vi "PopulateClearCycles.vi"(10 "ClearCycles":refnum<k24>, 11 "Digital in":refnum<vi>) -> ()   [LabVIEW 2019]
uses:
  Dependencies/PVCamNET.dll
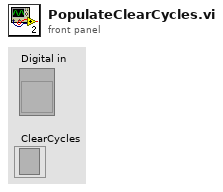
[diagram p1: front panel]
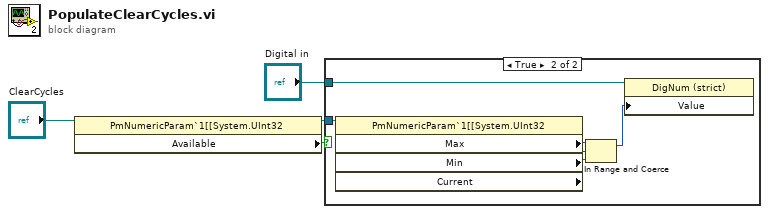
[diagram p0: block diagram]
diagram:
  n1 = property class="PmNumericParam`1[[System.UInt32"(reference="ClearCycles") -> (reference out=w3:refnum<k24>, "Available"=w2:bool)  [unwired: 1 in, 1 out]
  n2 = case shown="True" w2 {
    tunnel: w3 -> [_ w10]
    tunnel: "Digital in" -> [_ w5]
    frame False {
    }
    frame True {
      n3 = property class="PmNumericParam`1[[System.UInt32"(reference=w10) -> ("Max"=w9:u32, "Min"=w8:u32, "Current"=w7:u32)  [unwired: 1 in, 2 out]
      n4 = In Range and Coerce(upper limit=w9, x=w7, lower limit=w8) -> (coerced(x)=w6:u32)  [unwired: 1 out]
      n5 = property class="DigNum (strict)"(reference=w5, "Value"=w6) -> ()  [unwired: 1 in, 2 out]
    }
  }
